vi "SRT-2014-Controls-Full.vi"() -> ()   [LabVIEW 2013]
uses:
  <vilib>/DAQmx/write.llb/DAQmx Write (Digital Bool 1Line 1Point).vi
panel:
  out "He  Venting":bool
  in  "He  Vent":bool
  out "He Filling":bool
  in  "He Fill":bool
  out "ESTES Ignition":bool
  out "O2 Ignite":bool
  in  "O2 Ignite":bool
  out "O2 Dropped":bool
  out "O2 Filling":bool
  in  "O2 Fill":bool
  out "N2O Venting":bool
  out "N2O Filling":bool
  in  "Emergency Stop":bool
  in  "Disconnected":bool
  in  "Done W/ N2O":bool
  in  "O2 Drop":bool
  in  "N2O QD":bool
  in  "N2O Vent":bool
  in  "N2O Fill":bool
  # "Turns off ALL N20 Controls"
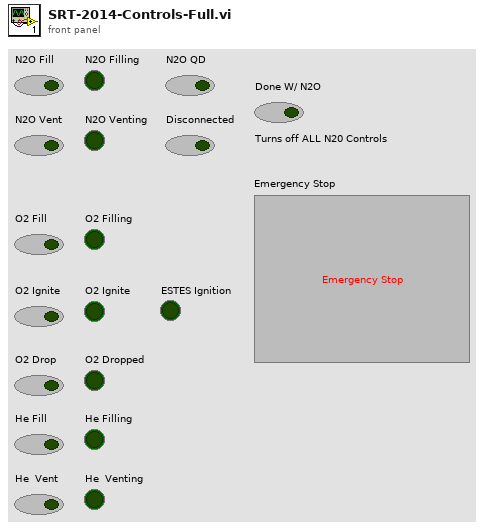
[diagram p1: front panel]
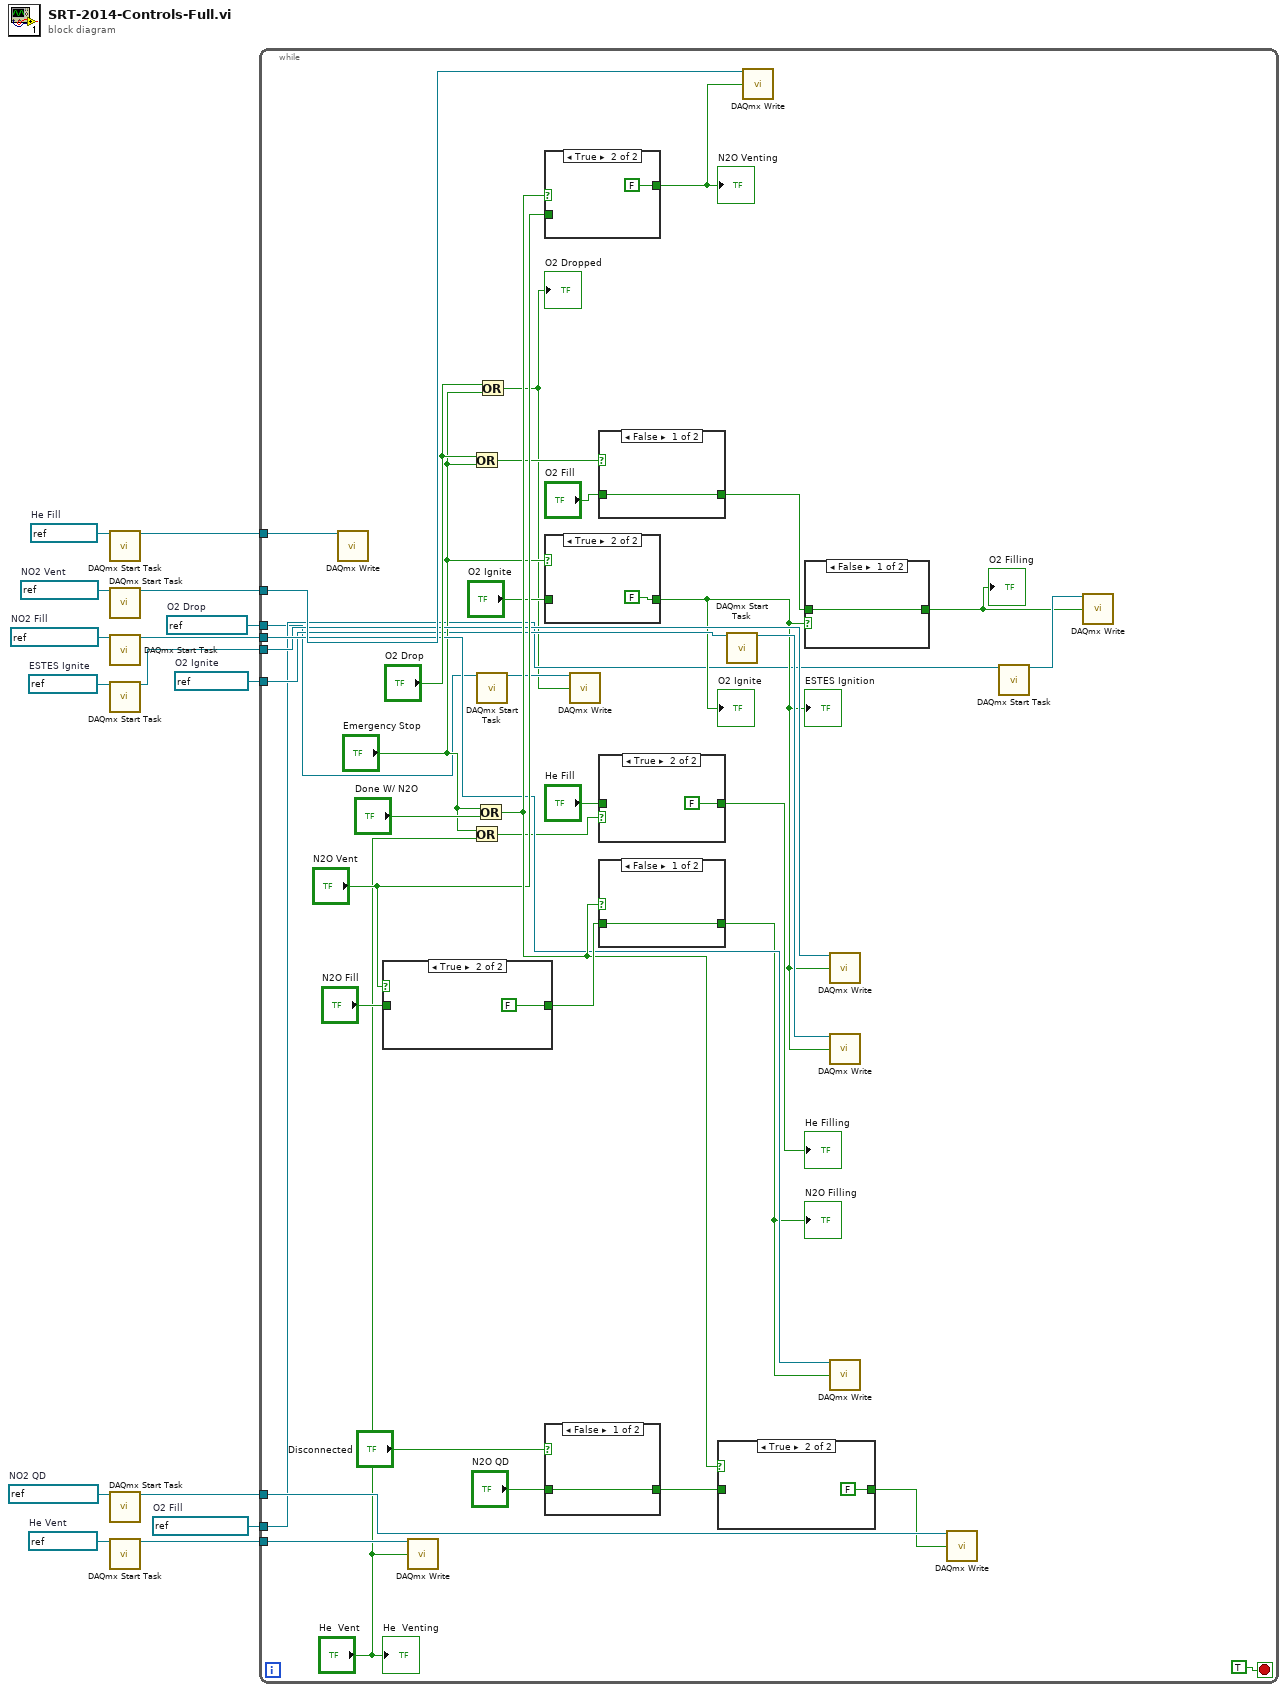
[diagram p0: block diagram]
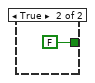
[diagram p3: hidden frame]
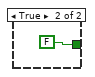
[diagram p5: hidden frame]
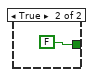
[diagram p7: hidden frame]
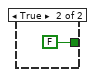
[diagram p9: hidden frame]
diagram:
  w6 = refnum<k21> refnum  # He Vent
  w7 = refnum<k21> refnum  # He Fill
  w9 = refnum<k21> "2_3"  # ESTES Ignite
  w13 = refnum<k21> "1_0"  # NO2 Fill
  w11 = refnum<k21> "1_2"  # NO2 QD
  w3 = refnum<k21> "2_3"  # O2 Ignite
  w2 = refnum<k21> "2_0"  # O2 Fill
  w1 = refnum<k21> "2_1"  # O2 Drop
  w15 = refnum<k21> "1_1"  # NO2 Vent
  n1 = call <vilib>:"DAQmx Start Task.vi"("task/channels in"=w7) -> ("task out"=w5:refnum<k21>)  [unwired: 13 in, 1 out]
  n2 = call <vilib>:"DAQmx Start Task.vi"("task/channels in"=w15) -> ("task out"=w14:refnum<k21>)  [unwired: 13 in, 1 out]
  n3 = call <vilib>:"DAQmx Start Task.vi"("task/channels in"=w13) -> ("task out"=w12:refnum<k21>)  [unwired: 13 in, 1 out]
  n4 = call <vilib>:"DAQmx Start Task.vi"("task/channels in"=w9) -> ("task out"=w8:refnum<k21>)  [unwired: 13 in, 1 out]
  n5 = call <vilib>:"DAQmx Start Task.vi"("task/channels in"=w11) -> ("task out"=w10:refnum<k21>)  [unwired: 13 in, 1 out]
  n6 = call <vilib>:"DAQmx Start Task.vi"("task/channels in"=w6) -> ("task out"=w4:refnum<k21>)  [unwired: 13 in, 1 out]
  n7 = while {
    tunnel: w14 -> [w39]
    tunnel: w12 -> [w37]
    tunnel: w10 -> [w35]
    tunnel: w8 -> [w33]
    tunnel: w5 -> [w31]
    tunnel: w4 -> [w30]
    tunnel: w3 -> [w24]
    tunnel: w2 -> [w21]
    tunnel: w1 -> [w18]
    stop <- TRUE stop-if-true
    n8 = call-poly <vilib>:"DAQmx Write.vi"("task/channels in"=w31) -> ()  [unwired: 12 in, 3 out]
    n9 = case shown="True" "N2O Vent" {
      tunnel: "N2O Fill" -> [w69 _]
      tunnel: [w69 FALSE] -> w50
      frame False {
      }
      frame True {
      }
    }
    n10 = call-poly <vilib>:"DAQmx Write.vi"("task/channels in"=w30, "data"="He  Vent") -> ()  [unwired: 11 in, 3 out]
    n11 = Or(x="O2 Drop", y="Emergency Stop") -> (x .or. y?=w42:bool)
    n12 = Or(x="Emergency Stop", y="He  Vent") -> (x .or. y?=w25:bool)
    n13 = Or(x="Emergency Stop", y="Done W/ N2O") -> (x .or. y?=w47:bool)
    n14 = call <vilib>:"DAQmx Start Task.vi"("task/channels in"=w18) -> ("task out"=w17:refnum<k21>)  [unwired: 13 in, 1 out]
    n15 = Or(x="O2 Drop", y="Emergency Stop") -> (x .or. y?=w16:bool)
    "O2 Dropped" <- w16
    n16 = case shown="True" w47 {
      tunnel: [w65 FALSE] -> w38
      tunnel: "N2O Vent" -> [w65 _]
      frame False {
      }
      frame True {
      }
    }
    "N2O Venting" <- w38
    n17 = case shown="True" "Emergency Stop" {
      tunnel: [w57 FALSE] -> w22
      tunnel: "O2 Ignite" -> [w57 _]
      frame False {
      }
      frame True {
      }
    }
    "O2 Ignite" <- w22
    "ESTES Ignition" <- w22
    n18 = case shown="False" "Disconnected" {
      tunnel: "N2O QD" -> [w67 _]
      tunnel: [w67 FALSE] -> w49
      frame False {
      }
      frame True {
      }
    }
    n19 = call-poly <vilib>:"DAQmx Write.vi"("task/channels in"=w17, "data"=w16) -> ()  [unwired: 11 in, 3 out]
    n20 = case shown="False" w42 {
      tunnel: [w59 FALSE] -> w32
      tunnel: "O2 Fill" -> [w59 _]
      frame False {
      }
      frame True {
      }
    }
    n21 = case shown="True" w25 {
      tunnel: "He Fill" -> [w53 _]
      tunnel: [w53 FALSE] -> w28
      frame False {
      }
      frame True {
      }
    }
    "He Filling" <- w28
    n22 = case shown="False" w47 {
      tunnel: w50 -> [w63 _]
      tunnel: [w63 FALSE] -> w36
      frame False {
      }
      frame True {
      }
    }
    "N2O Filling" <- w36
    n23 = case shown="True" w47 {
      tunnel: w49 -> [w61 _]
      tunnel: [w61 FALSE] -> w34
      frame False {
      }
      frame True {
      }
    }
    n24 = call <vilib>:"DAQmx Start Task.vi"("task/channels in"=w24) -> ("task out"=w23:refnum<k21>)  [unwired: 13 in, 1 out]
    n25 = call-poly <vilib>:"DAQmx Write.vi"("task/channels in"=w39, "data"=w38) -> ()  [unwired: 11 in, 3 out]
    n26 = case shown="False" w22 {
      tunnel: [w55 FALSE] -> w19
      tunnel: w32 -> [w55 _]
      frame False {
      }
      frame True {
      }
    }
    "O2 Filling" <- w19
    n27 = call-poly <vilib>:"DAQmx Write.vi"("task/channels in"=w33, "data"=w22) -> ()  [unwired: 11 in, 3 out]
    n28 = call-poly <vilib>:"DAQmx Write.vi"("task/channels in"=w23, "data"=w22) -> ()  [unwired: 11 in, 3 out]
    n29 = call-poly <vilib>:"DAQmx Write.vi"("task/channels in"=w37, "data"=w36) -> ()  [unwired: 11 in, 3 out]
    n30 = call-poly <vilib>:"DAQmx Write.vi"("task/channels in"=w35, "data"=w34) -> ()  [unwired: 11 in, 3 out]
    n31 = call <vilib>:"DAQmx Start Task.vi"("task/channels in"=w21) -> ("task out"=w20:refnum<k21>)  [unwired: 13 in, 1 out]
    n32 = call-poly <vilib>:"DAQmx Write.vi"("task/channels in"=w20, "data"=w19) -> ()  [unwired: 11 in, 3 out]
    "He  Venting" <- "He  Vent"
  }
